vi "Filter Wheel Update Status.vi"(8 "error in (no error)":errorcluster, 11 "FW Status":T1={"State"=enum."Move Complete", "Positions"=[], "Names"=[], "Notch"=[], "Moving"=[FALSE, FALSE]}) -> (0 "error out":errorcluster)   [LabVIEW 2024]
uses:
  FW cluster Status.ctl
  FW enum status.ctl
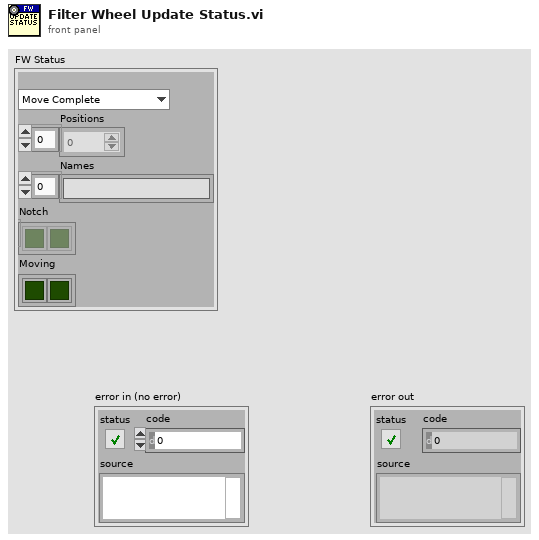
[diagram p1: front panel]
types:
  T1 = typedef "FW cluster Status.ctl" = cluster{"State":T2, "Positions":i32[], "Names":string[], "Notch":bool[], "Moving":bool[]}
  T2 = typedef "FW enum status.ctl" = enum16{"Initializing", "Moving", "Move Complete", "Error"}
  T3 = typedef "CC Current Status.ctl" = cluster{"Target":string, "Filter 1":string, "Filter 2":string}
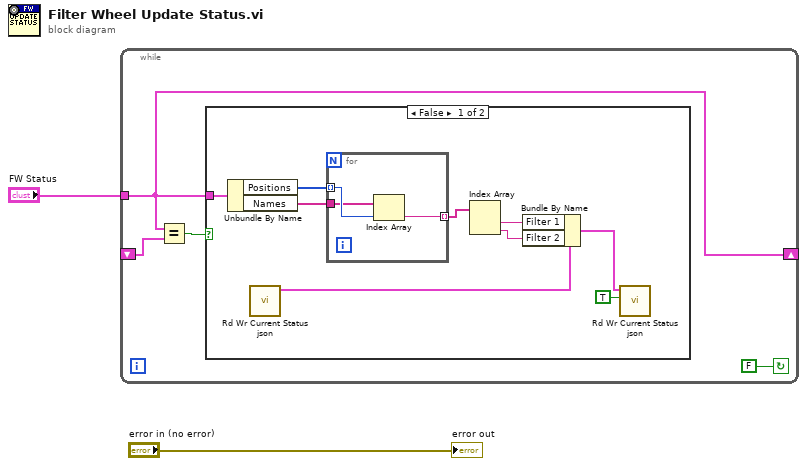
[diagram p0: block diagram]
diagram:
  n1 = while {
    tunnel: "FW Status" -> [w5]
    shift-right: [w5] -> _
    shift-left: _ -> [w4]
    stop <- FALSE continue-if-true
    n2 = Equal?(x=w5, y=w4) -> (x = y?=w3:bool)
    n3 = case shown="False" w3 {
      tunnel: w5 -> [w13 _]
      frame False {
        n4 = Unbundle By Name(w13) -> ("Positions"=w15:i32[], "Names"=w14:string[])
        n5 = call "Rd Wr Current Status json.vi"() -> ("Current Status"=w12:T3)  [unwired: 10 in, 1 out]
        n6 = for {
          tunnel: w15 -> [w18] mode=indexing
          tunnel: w14 -> [w17]
          tunnel: [w16] -> w11 mode=indexing
          n7 = Index Array(array=w17, index=w18) -> (element=w16:string)
        }
        n8 = Index Array(array=w11) -> (element #1=w10:string, element #2=w9:string)  [unwired: 2 in]
        n9 = Bundle By Name(cluster=w12, "Filter 1"=w10, "Filter 2"=w9) -> (w8:T3)
        n10 = call "Rd Wr Current Status json.vi"("Write? (F:Read)"=TRUE, "Current Status"=w8) -> ()  [unwired: 8 in, 2 out]
      }
      frame True {
      }
    }
  }
  "error out" <- "error in (no error)"
